vi "Motor.vi"(8 "error in (no error)":errorcluster, 9 "Command [-5 5]":dbl min=-1.0 max=1.0 step=0.01, 10 "Enable":bool=TRUE) -> (0 "error out":errorcluster)   [LabVIEW 2019]
uses:
  <vilib>/myRIO/Instrument Drivers/Onboard IO/DIO/typedefs/DIO Reference.ctl
  <vilib>/myRIO/Common/Instrument Driver Framework/Utilities/typedefs/myRIO Generic Hardware Reference.ctl
  <vilib>/myRIO/Common/Instrument Driver Framework/Utilities/typedefs/Hardware Version Enum.ctl
  <vilib>/myRIO/Common/Instrument Driver Framework/Utilities/typedefs/myRIO v1.0 Reference.ctl
  <vilib>/myRIO/Common/Instrument Driver Framework/Utilities/typedefs/Generic FPGA Reference.ctl
  <vilib>/myRIO/Common/Instrument Driver Framework/myRIO v1.0/DIO/typedefs/DIO Channels List.ctl
  <vilib>/myRIO/Common/Instrument Driver Framework/myRIO v1.0/DIO/typedefs/DIO Channels Enum.ctl
  <vilib>/userdefined/High Color/nirio_resource_hc.ctl
  <vilib>/myRIO/Instrument Drivers/Onboard IO/PWM/typedefs/PWM Reference.ctl
  <vilib>/myRIO/Common/Instrument Driver Framework/myRIO v1.0/PWM/typedefs/PWM Channels Enum.ctl
  <vilib>/myRIO/Instrument Drivers/Onboard IO/PWM/typedefs/PWM Configuration.ctl
  <vilib>/myRIO/Common/Instrument Driver Framework/Utilities/vis/Is FPGA Ref Available.vi
  <vilib>/myRIO/Common/Instrument Driver Framework/ELVIS III v1.0/DIO/vis/ELVIS III v1.1 Open DIO.vi
  <vilib>/myRIO/Instrument Drivers/Onboard IO/DIO/vis/Write.vi
  <vilib>/myRIO/Common/Instrument Driver Framework/ELVIS III v1.0/PWM/vis/ELVIS III v1.1 Open PWM.vi
  <vilib>/myRIO/Instrument Drivers/Onboard IO/PWM/vis/Set Duty Cycle and Frequency.vi
  <vilib>/myRIO/Common/Instrument Driver Framework/Utilities/vis/Validate Channels.vi
  <vilib>/myRIO/Common/Instrument Driver Framework/ELVIS III v1.0/DIO/vis/ELVIS III v1.0 Reserve DIO.vi
  <vilib>/myRIO/Common/Instrument Driver Framework/ELVIS III v1.0/PWM/vis/ELVIS III v1.0 Reserve PWM.vi
  <vilib>/myRIO/Common/Instrument Driver Framework/ELVIS III v1.0/DIO/vis/ELVIS III v1.0 Build MUX Configuration DIO.vi
  <vilib>/myRIO/Common/Instrument Driver Framework/ELVIS III v1.0/PWM/vis/ELVIS III v1.0 Build MUX Configuration PWM.vi
  <vilib>/myRIO/Common/Instrument Driver Framework/ELVIS III v1.0/Resource Manager/vis/ELVIS III v1.0 Create Configuration List.vi
  <vilib>/Utility/VariantDataType/GetNumericInfo.vi
  <vilib>/Utility/error.llb/Error Cluster From Error Code.vi
  <vilib>/myRIO/Common/Instrument Driver Framework/ELVIS III v1.0/ELVIS III v1.1 Open.vi
  <vilib>/myRIO/Common/Instrument Driver Framework/ELVIS III v1.0/Resource Manager/vis/ELVIS III v1.0 Reserve Channel List.vi
  <vilib>/myRIO/Common/Instrument Driver Framework/ELVIS III v1.0/Resource Manager/vis/ELVIS III v1.0 Configure IO.vi
  <vilib>/myRIO/Common/Instrument Driver Framework/myRIO v1.0/myRIO v1.0 Close.vi
  <vilib>/myRIO/Common/Instrument Driver Framework/ELVIS III v1.0/DIO/vis/ELVIS III v1.0 Write DIO.vi
  <vilib>/myRIO/Common/Instrument Driver Framework/ELVIS III v1.0/PWM/vis/ELVIS III v1.0 Write PWM.vi
  <vilib>/myRIO/Express VI/Onboard IO/DO/DO Express VI.xnode
  <vilib>/myRIO/Instrument Drivers/Onboard IO/DIO/vis/myRIO DIO Open.xnode
  <vilib>/myRIO/Express VI/Onboard IO/PWM/PWM Express VI.xnode
  <vilib>/myRIO/Instrument Drivers/Onboard IO/PWM/vis/myRIO PWM Open.xnode
  <vilib>/myRIO/Instrument Drivers/Onboard IO/DIO/DIO.lvlib
  <vilib>/myRIO/Instrument Drivers/Onboard IO/PWM/PWM.lvlib
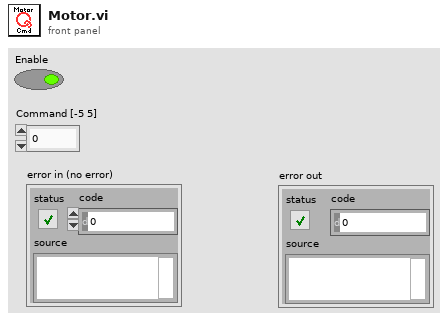
[diagram p1: front panel]
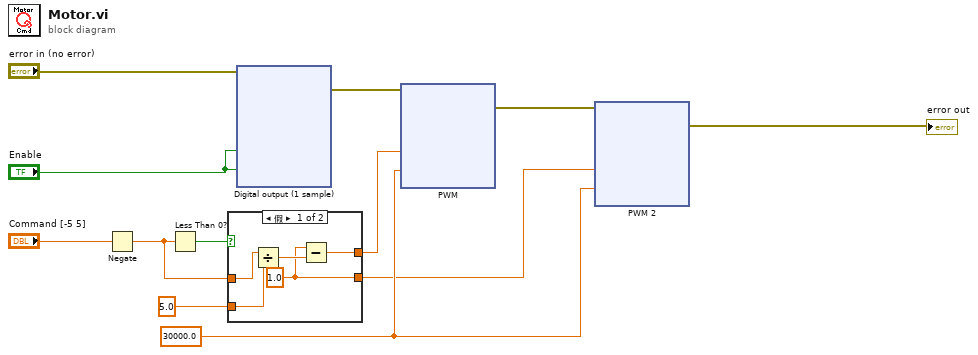
[diagram p0: block diagram]
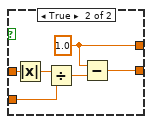
[diagram p2: hidden frame]
diagram:
  w9 = 30000.0 ("Frequency [Hz]")
  n1 = Negate(x="Command [-5 5]") -> (-x=w2:dbl)
  n2 = Less Than 0?(x=w2) -> (x < 0?=w8:bool)
  n3 = case shown="假" w8 {
    tunnel: w2 -> [w17 w23]
    tunnel: [w13 w20] -> w6
    tunnel: [w14 w19] -> w7
    tunnel: 5.0 -> [w16 w21]
    frame False {
      w13 = 1.0
      n4 = Divide(x=w17, y=w16) -> (x/y=w15:dbl)
      n5 = Subtract(x=w13, y=w15) -> (x-y=w14:dbl)
    }
    frame True {
      w19 = 1.0
      n6 = Absolute Value(x=w23) -> (abs(x)=w22:dbl)
      n7 = Divide(x=w22, y=w21) -> (x/y=w18:dbl)
      n8 = Subtract(x=w19, y=w18) -> (x-y=w20:dbl)
    }
  }
  n9 = xnode "Digital output (1 sample)"("A/DIO19 (Pin 115)"="Enable", "B/DIO17 (Pin 133)"="Enable", "error in (no error)"="error in (no error)") -> ("error out"=w11:errorcluster)
  n10 = xnode "PWM"("Duty Cycle"=w7, "Frequency [Hz]"=w9, "error in (no error)"=w11) -> ("error out"=w10:errorcluster)
  n11 = xnode "PWM 2"("Duty Cycle"=w6, "Frequency [Hz]"=w9, "error in (no error)"=w10) -> ("error out"=→"error out":errorcluster)
